vi "Handler - FPGA Health Alert.vi"(8 "error in (no error)":errorcluster, 11 "FPGA Health Info":T1) -> (0 "error out":errorcluster, 3 "Exit?":bool)   [LabVIEW 2018]
uses:
  Top Level/Shared Controls/FPGA Alert Info.ctl
  Error Handler.lvlib
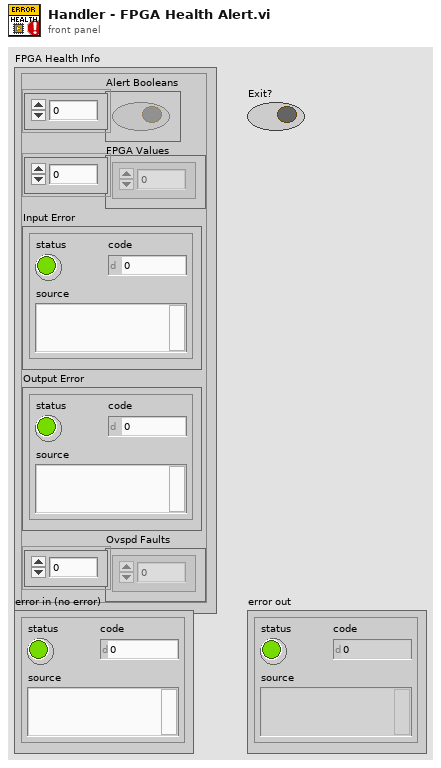
[diagram p1: front panel]
types:
  T1 = typedef "FPGA Alert Info.ctl" = cluster{"Alert Booleans":bool[], "FPGA Values":u64[], "Input Error":errorcluster, "Output Error":errorcluster, "Ovspd Faults":sgl[]}
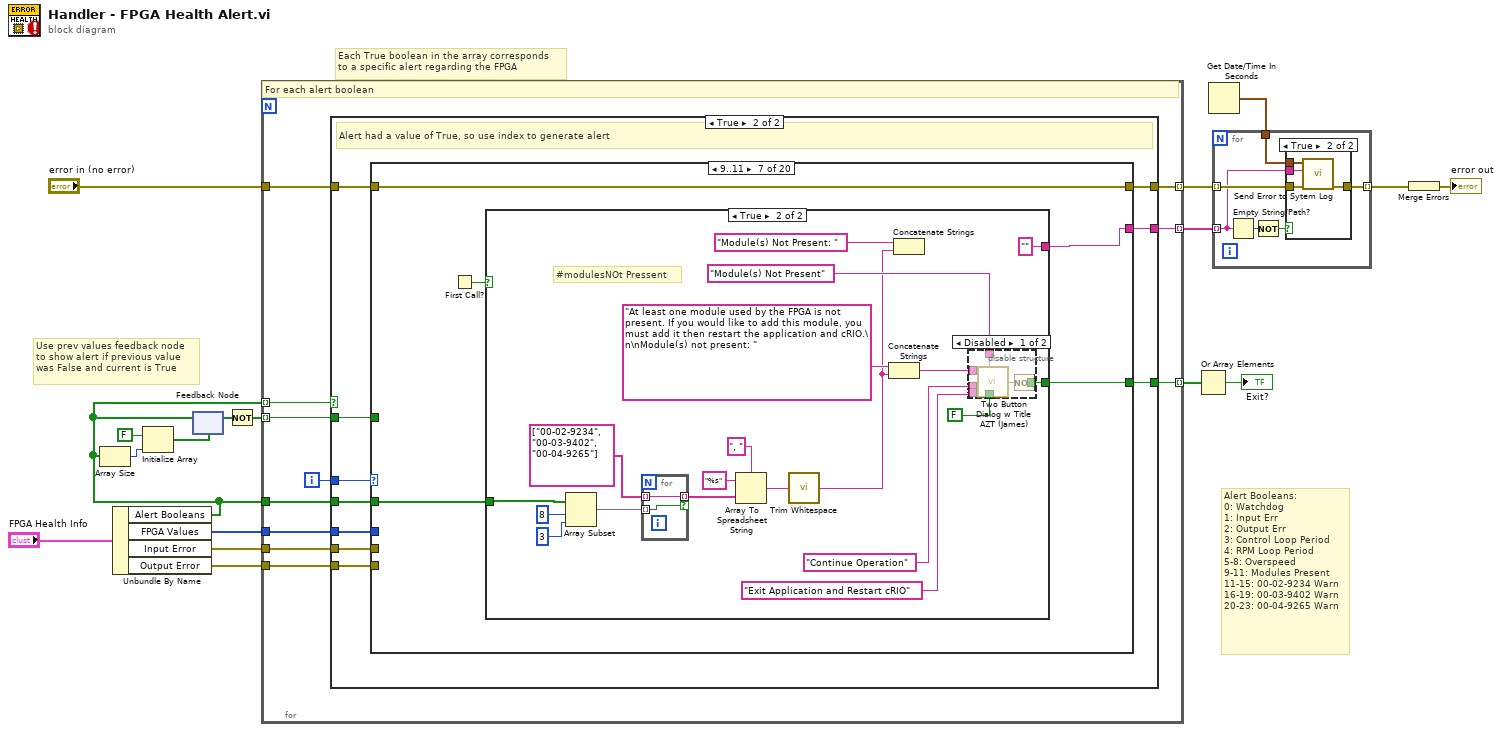
[diagram p0: block diagram]
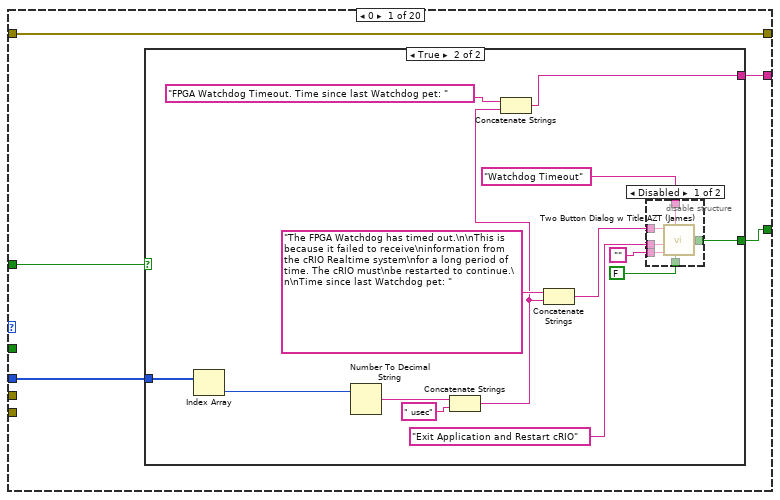
[diagram p4: hidden frame]
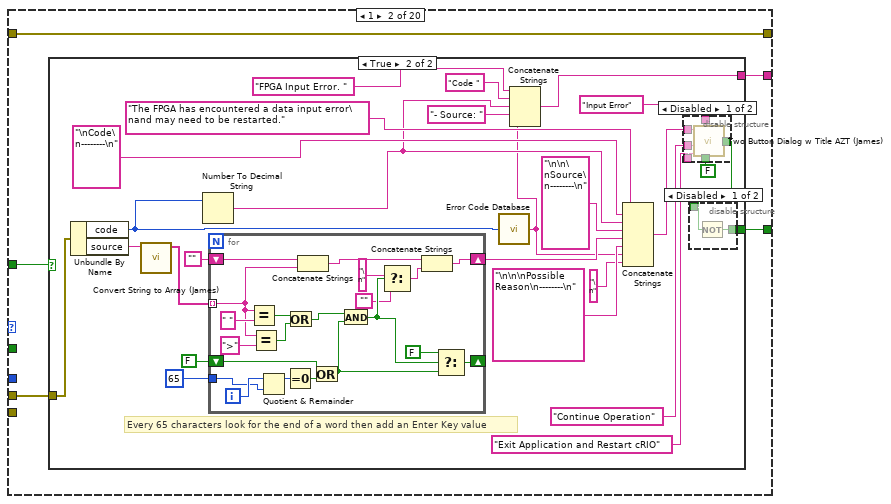
[diagram p7: hidden frame]
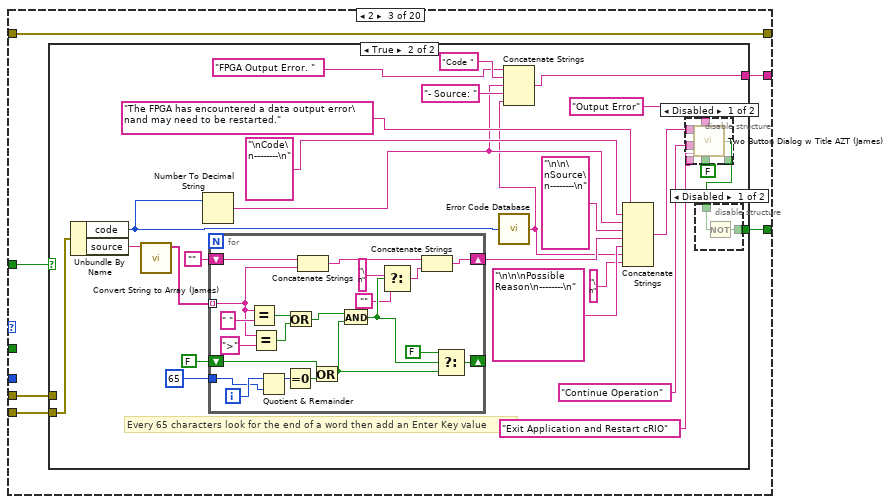
[diagram p11: hidden frame]
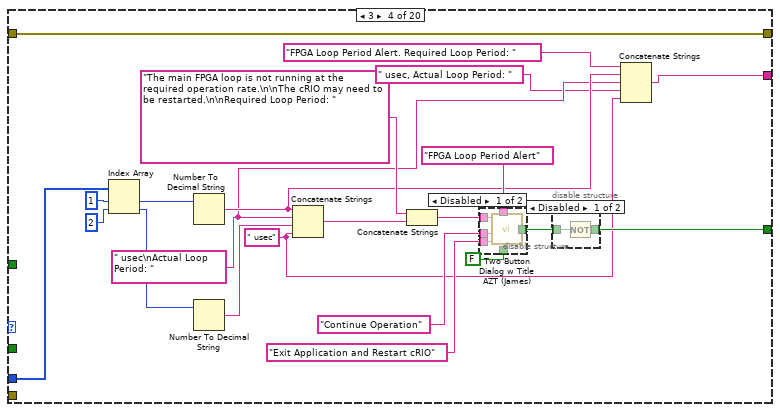
[diagram p15: hidden frame]
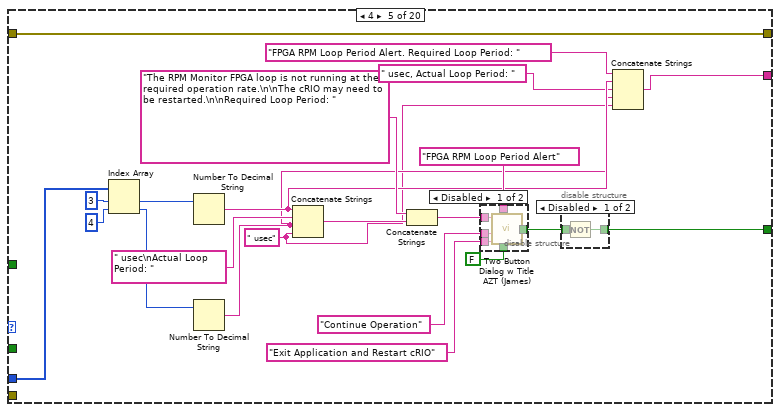
[diagram p18: hidden frame]
diagram:
  # "Alert Booleans:\n0: Watchdog\n1: Input Err\n2: Output Err\n3: Control Loop Period\n4: RPM Loop Period\n5-8: Overspeed\n9-11: Modules Present\n11-15: 00-02-9234 Warn\n16-19: 00-03-9402 Warn\n20-23: 00-04-9265 Warn"
  # "Use prev values feedback node\nto show alert if previous value\nwas False and current is True"
  # "Each True boolean in the array corresponds\nto a specific alert regarding the FPGA"
  n1 = Unbundle By Name("FPGA Health Info") -> ("Alert Booleans"=w9:bool[], "FPGA Values"=w15:u64[], "Input Error"=w12:errorcluster, "Output Error"=w11:errorcluster)
  n2 = Array Size(array=w9) -> (size(s)=w8:i32)
  n3 = Initialize Array(FALSE, w8) -> (w7:bool[])
  n4 = feedback #1(w7) -> (w6:bool[])
  n5 = feedback-in #1(w9) -> ()
  n6 = Not(x=w6) -> (.not. x?=w5:bool[])
  n7 = for {
    tunnel: w9 -> [w28] mode=indexing
    tunnel: "error in (no error)" -> [w26]
    tunnel: [w27] -> w4 mode=indexing
    tunnel: w15 -> [w25]
    tunnel: [w24] -> w16 mode=indexing
    tunnel: w12 -> [w23]
    tunnel: w11 -> [w22]
    tunnel: w9 -> [w21]
    tunnel: w5 -> [w20] mode=indexing
    tunnel: [w19] -> w2 mode=indexing
    i -> [w29]
    # "For each alert boolean"
    n8 = case shown="True" w28 {
      tunnel: w29 -> [_ w40]
      tunnel: [w30 w38] -> w27
      tunnel: w26 -> [w30 w39]
      tunnel: w25 -> [_ w37]
      tunnel: [_ w36] -> w24
      tunnel: w23 -> [_ w35]
      tunnel: w22 -> [_ w34]
      tunnel: w21 -> [_ w33]
      tunnel: w20 -> [_ w32]
      tunnel: [_ w31] -> w19
      frame False {
      }
      frame True {
        # "Alert had a value of True, so use index to generate alert"
        n9 = case shown="9..11" w40 {
          selector: w40 -> [_ _ _ _ _ w249 _ _ _ _ _ _ _ _ _ _ _ _ _ w538]
          tunnel: w39 -> [w45 w70 w131 w207 w237 w251 w278 w309 w328 w347 w366 w385 w404 w423 w442 w462 w481 w501 w520 w545]
          tunnel: [w45 w70 w131 w207 w237 w251 w278 w309 w328 w347 w366 w385 w404 w423 w442 w462 w481 w501 w520 w545] -> w38
          tunnel: w37 -> [w43 _ _ w203 w233 _ _ _ _ _ _ _ _ _ _ _ _ _ _ _]
          tunnel: [w44 w69 w130 w194 w223 w250 w277 w308 w327 w346 w365 w384 w403 w422 w441 w461 w480 w500 w519 _] -> w36
          tunnel: w35 -> [_ w68 w129 _ _ _ _ _ _ _ _ _ _ _ _ _ _ _ _ _]
          tunnel: w34 -> [_ _ w128 _ _ _ _ _ _ _ _ _ _ _ _ _ _ _ _ _]
          tunnel: w33 -> [_ _ _ _ _ _ w275 _ _ _ _ _ _ _ _ _ _ _ _ _]
          tunnel: w32 -> [w42 w67 w127 _ _ w248 _ w307 w326 w345 w364 w383 w402 w421 w440 w460 w479 w499 w518 _]
          tunnel: [w41 w66 w126 w191 w217 w247 w274 _ _ _ _ _ _ _ _ w459 w478 _ _ _] -> w31
          frame 0 {
            n10 = case shown="True" w42 {
              tunnel: [_ w56] -> w44
              tunnel: w43 -> [_ w55]
              tunnel: [_ w46] -> w41
              frame False {
              }
              frame True {
                n11 = Index Array(array=w55) -> (element=w54:u64)  [unwired: 1 in]
                n12 = Number To Decimal String(number=w54) -> (decimal integer string=w53:string)  [unwired: 1 in]
                n13 = Concatenate Strings(w53, " usec" ("string")) -> (w47:string)
                n14 = Concatenate Strings("FPGA Watchdog Timeout. Time since last Watchdog pet: " ("Window Title (\"\")"), w47) -> (w46:string)
                n15 = Concatenate Strings("The FPGA Watchdog has timed out.\n\nThis is because it failed to receive\ninformation from the cRIO Realtime system\nfor a long period of time. The cRIO must\nbe restarted to continue.\n\nTime since last Watchdog pet: " ("message"), w47) -> (w57:string)
                n16 = disable-structure shown="Disabled" {
                  disable-tunnel: "Watchdog Timeout" ("Window Title (\"\")") -> [w65 _]
                  disable-tunnel: w57 -> [w64 _]
                  disable-tunnel: [w63 _] -> w56
                  disable-tunnel: FALSE ("Allow user to close window? (TRUE)") -> [w62 _]
                  disable-tunnel: "Exit Application and Restart cRIO" ("T button name (\"OK\")") -> [w61 _]
                  disable-tunnel: "" -> [w60 _]
                  frame Disabled {
                    n17 = call "Two Button Dialog w Title AZT (James).vi"("Allow user to close window? (TRUE)"=w62, "Window Title (\"\")"=w65, "F button name (\"Cancel\")"=w60, "T button name (\"OK\")"=w61, "message"=w64) -> ("T Button?"=w63:bool)  [unwired: 1 in]
                  }
                  frame Enabled {
                  }
                }
              }
            }
          }
          frame 1 {
            n18 = case shown="True" w67 {
              tunnel: [_ w79] -> w69
              tunnel: w68 -> [_ w82]
              tunnel: [_ w72] -> w66
              frame False {
              }
              frame True {
                # "Every 65 characters look for the end of a word then add an Enter Key value"
                n19 = Unbundle By Name(w82) -> ("code"=w91:i32, "source"=w73:string)
                n20 = call "Convert String to Array (James).vi"("String in"=w73) -> ("Array out"=w88:string[])  [unwired: 9 in, 1 out]
                n21 = Number To Decimal String(number=w91) -> (decimal integer string=w74:string)  [unwired: 1 in]
                n22 = for {
                  tunnel: w88 -> [w119] mode=indexing
                  shift-right: [w116] -> w86
                  shift-left: "" -> [w124]
                  tunnel: 65 ("length") -> [w105]
                  shift-right: [w114] -> _
                  shift-left: FALSE -> [w110]
                  i -> [w106]
                  n23 = Equal?(x=w119, y=" ") -> (x = y?=w120:bool)
                  n24 = Equal?(x=w119, y=">") -> (x = y?=w117:bool)
                  n25 = Quotient & Remainder(x=w106, y=w105) -> (x-y*floor(x/y)=w123:i32)  [unwired: 1 out]
                  n26 = Equal To 0?(x=w123) -> (x = 0?=w122:bool)
                  n27 = Or(x=w120, y=w117) -> (x .or. y?=w111:bool)
                  n28 = Concatenate Strings(w124, w119) -> (w125:string)
                  n29 = Or(x=w110, y=w122) -> (x .or. y?=w109:bool)
                  n30 = And(x=w111, y=w109) -> (x .and. y?=w115:bool)
                  n31 = Select(t="\n", s=w115, f="") -> (s? t:f=w112:string)
                  n32 = Concatenate Strings(w125, w112) -> (w116:string)
                  n33 = Select(t=FALSE, s=w115, f=w109) -> (s? t:f=w114:bool)
                }
                n34 = call <vilib>:"Error Code Database.vi"("Error Code"=w91) -> ("Error Text"=w71:string)
                n35 = Concatenate Strings("FPGA Input Error. " ("Window Title (\"\")"), "Code " ("string"), w74, "- Source: " ("string"), w71) -> (w72:string)
                n36 = Concatenate Strings("The FPGA has encountered a data input error\nand may need to be restarted." ("message"), "\nCode\n--------\n", w74, "\n\n\nSource\n--------\n", w86, "\n\n\nPossible Reason\n--------\n" ("string"), w71, "\n" ("string")) -> (w78:string)
                n37 = disable-structure shown="Disabled" {
                  disable-tunnel: "Input Error" ("Window Title (\"\")") -> [w104 _]
                  disable-tunnel: [w103 _] -> w95
                  disable-tunnel: FALSE ("Allow user to close window? (TRUE)") -> [w102 _]
                  disable-tunnel: w78 -> [w101 _]
                  disable-tunnel: "Continue Operation" ("F button name (\"Cancel\")") -> [w100 _]
                  disable-tunnel: "Exit Application and Restart cRIO" ("T button name (\"OK\")") -> [w99 _]
                  frame Disabled {
                    n38 = call "Two Button Dialog w Title AZT (James).vi"("Allow user to close window? (TRUE)"=w102, "Window Title (\"\")"=w104, "F button name (\"Cancel\")"=w99, "T button name (\"OK\")"=w100, "message"=w101) -> ("T Button?"=w103:bool)  [unwired: 1 in]
                  }
                  frame Enabled {
                  }
                }
                n39 = disable-structure shown="Disabled" {
                  disable-tunnel: w95 -> [w98 _]
                  disable-tunnel: [w97 _] -> w79
                  frame Disabled {
                    n40 = Not(x=w98) -> (.not. x?=w97:bool)
                  }
                  frame Enabled {
                  }
                }
              }
            }
          }
          frame 2 {
            n41 = case shown="True" w127 {
              tunnel: [_ w140] -> w130
              tunnel: w129 -> [_ _]
              tunnel: w128 -> [_ w143]
              tunnel: [_ w136] -> w126
              frame False {
              }
              frame True {
                # "Every 65 characters look for the end of a word then add an Enter Key value"
                n42 = Unbundle By Name(w143) -> ("code"=w152:i32, "source"=w133:string)
                n43 = call "Convert String to Array (James).vi"("String in"=w133) -> ("Array out"=w149:string[])  [unwired: 9 in, 1 out]
                n44 = Number To Decimal String(number=w152) -> (decimal integer string=w134:string)  [unwired: 1 in]
                n45 = for {
                  tunnel: w149 -> [w180] mode=indexing
                  shift-right: [w177] -> w147
                  shift-left: "" -> [w185]
                  tunnel: 65 ("length") -> [w166]
                  shift-right: [w175] -> _
                  shift-left: FALSE -> [w171]
                  i -> [w167]
                  n46 = Equal?(x=w180, y=" ") -> (x = y?=w181:bool)
                  n47 = Equal?(x=w180, y=">") -> (x = y?=w178:bool)
                  n48 = Quotient & Remainder(x=w167, y=w166) -> (x-y*floor(x/y)=w184:i32)  [unwired: 1 out]
                  n49 = Equal To 0?(x=w184) -> (x = 0?=w183:bool)
                  n50 = Or(x=w181, y=w178) -> (x .or. y?=w172:bool)
                  n51 = Concatenate Strings(w185, w180) -> (w186:string)
                  n52 = Or(x=w171, y=w183) -> (x .or. y?=w170:bool)
                  n53 = And(x=w172, y=w170) -> (x .and. y?=w176:bool)
                  n54 = Select(t="\n", s=w176, f="") -> (s? t:f=w173:string)
                  n55 = Concatenate Strings(w186, w173) -> (w177:string)
                  n56 = Select(t=FALSE, s=w176, f=w170) -> (s? t:f=w175:bool)
                }
                n57 = call <vilib>:"Error Code Database.vi"("Error Code"=w152) -> ("Error Text"=w132:string)
                n58 = Concatenate Strings("FPGA Output Error. " ("Window Title (\"\")"), "Code " ("string"), w134, "- Source: " ("string"), w132) -> (w136:string)
                n59 = Concatenate Strings("The FPGA has encountered a data output error\nand may need to be restarted." ("message"), "\nCode\n--------\n", w134, "\n\n\nSource\n--------\n", w147, "\n\n\nPossible Reason\n--------\n" ("string"), w132, "\n" ("string")) -> (w139:string)
                n60 = disable-structure shown="Disabled" {
                  disable-tunnel: "Output Error" ("Window Title (\"\")") -> [w165 _]
                  disable-tunnel: [w164 _] -> w156
                  disable-tunnel: FALSE ("Allow user to close window? (TRUE)") -> [w163 _]
                  disable-tunnel: w139 -> [w162 _]
                  disable-tunnel: "Continue Operation" ("F button name (\"Cancel\")") -> [w161 _]
                  disable-tunnel: "Exit Application and Restart cRIO" ("T button name (\"OK\")") -> [w160 _]
                  frame Disabled {
                    n61 = call "Two Button Dialog w Title AZT (James).vi"("Allow user to close window? (TRUE)"=w163, "Window Title (\"\")"=w165, "F button name (\"Cancel\")"=w160, "T button name (\"OK\")"=w161, "message"=w162) -> ("T Button?"=w164:bool)  [unwired: 1 in]
                  }
                  frame Enabled {
                  }
                }
                n62 = disable-structure shown="Disabled" {
                  disable-tunnel: w156 -> [w159 _]
                  disable-tunnel: [w158 _] -> w140
                  frame Disabled {
                    n63 = Not(x=w159) -> (.not. x?=w158:bool)
                  }
                  frame Enabled {
                  }
                }
              }
            }
          }
          frame 3 {
            w189 = " usec" ("string")
            w190 = " usec\nActual Loop Period: " ("string")
            n64 = Index Array(array=w203, index #1=1 ("index"), index #2=2 ("index")) -> (element #1=w198:u64, element #2=w197:u64)
            n65 = Number To Decimal String(number=w198) -> (decimal integer string=w192:string)  [unwired: 1 in]
            n66 = Number To Decimal String(number=w197) -> (decimal integer string=w188:string)  [unwired: 1 in]
            n67 = Concatenate Strings(w192, w190, w188, w189) -> (w201:string)
            n68 = Concatenate Strings("The main FPGA loop is not running at the required operation rate.\n\nThe cRIO may need to be restarted.\n\nRequired Loop Period: " ("message"), w201) -> (w205:string)
            n69 = disable-structure shown="Disabled" {
              disable-tunnel: "FPGA Loop Period Alert" ("Window Title (\"\")") -> [w216 _]
              disable-tunnel: w205 -> [w215 _]
              disable-tunnel: [w214 _] -> w204
              disable-tunnel: FALSE ("Allow user to close window? (TRUE)") -> [w213 _]
              disable-tunnel: "Continue Operation" ("F button name (\"Cancel\")") -> [w212 _]
              disable-tunnel: "Exit Application and Restart cRIO" ("T button name (\"OK\")") -> [w211 _]
              frame Disabled {
                n70 = call "Two Button Dialog w Title AZT (James).vi"("Allow user to close window? (TRUE)"=w213, "Window Title (\"\")"=w216, "F button name (\"Cancel\")"=w211, "T button name (\"OK\")"=w212, "message"=w215) -> ("T Button?"=w214:bool)  [unwired: 1 in]
              }
              frame Enabled {
              }
            }
            n71 = disable-structure shown="Disabled" {
              disable-tunnel: w204 -> [w210 _]
              disable-tunnel: [w209 _] -> w194
              frame Disabled {
                n72 = Not(x=w210) -> (.not. x?=w209:bool)
              }
              frame Enabled {
              }
            }
            n73 = Concatenate Strings("FPGA Loop Period Alert. Required Loop Period: " ("Window Title (\"\")"), w192, w190, " usec, Actual Loop Period: " ("string"), w189) -> (w191:string)
          }
          frame 4 {
            w218 = " usec" ("string")
            n74 = Index Array(array=w233, index #1=3 ("index"), index #2=4 ("index")) -> (element #1=w228:u64, element #2=w227:u64)
            n75 = Number To Decimal String(number=w228) -> (decimal integer string=w221:string)  [unwired: 1 in]
            n76 = Number To Decimal String(number=w227) -> (decimal integer string=w219:string)  [unwired: 1 in]
            n77 = Concatenate Strings(w221, " usec\nActual Loop Period: " ("string"), w219, w218) -> (w231:string)
            n78 = Concatenate Strings("The RPM Monitor FPGA loop is not running at the required operation rate.\n\nThe cRIO may need to be restarted.\n\nRequired Loop Period: " ("message"), w231) -> (w235:string)
            n79 = disable-structure shown="Disabled" {
              disable-tunnel: "FPGA RPM Loop Period Alert" ("Window Title (\"\")") -> [w246 _]
              disable-tunnel: w235 -> [w245 _]
              disable-tunnel: [w244 _] -> w234
              disable-tunnel: FALSE ("Allow user to close window? (TRUE)") -> [w243 _]
              disable-tunnel: "Continue Operation" ("F button name (\"Cancel\")") -> [w242 _]
              disable-tunnel: "Exit Application and Restart cRIO" ("T button name (\"OK\")") -> [w241 _]
              frame Disabled {
                n80 = call "Two Button Dialog w Title AZT (James).vi"("Allow user to close window? (TRUE)"=w243, "Window Title (\"\")"=w246, "F button name (\"Cancel\")"=w241, "T button name (\"OK\")"=w242, "message"=w245) -> ("T Button?"=w244:bool)  [unwired: 1 in]
              }
              frame Enabled {
              }
            }
            n81 = disable-structure shown="Disabled" {
              disable-tunnel: w234 -> [w240 _]
              disable-tunnel: [w239 _] -> w223
              frame Disabled {
                n82 = Not(x=w240) -> (.not. x?=w239:bool)
              }
              frame Enabled {
              }
            }
            n83 = Concatenate Strings("FPGA RPM Loop Period Alert. Required Loop Period: " ("Window Title (\"\")"), w221, " usec, Actual Loop Period: " ("string"), w219, w218) -> (w217:string)
          }
          frame 5..8 {
            n84 = case shown="True" w248 {
              tunnel: [_ w255] -> w250
              tunnel: w249 -> [_ w259]
              tunnel: [_ w252] -> w247
              frame False {
              }
              frame True {
                n85 = Subtract(x=w259, y=4) -> (x-y=w260:i32)
                n86 = Number To Decimal String(number=w260) -> (decimal integer string=w253:string)  [unwired: 1 in]
                n87 = Concatenate Strings("The FPGA has indicated an Overspeed Fault.\n\nFault Index: " ("message"), w253) -> (w263:string)
                n88 = Concatenate Strings("Overspeed Fault. Fault Index: " ("Window Title (\"\")"), w253) -> (w252:string)
                n89 = disable-structure shown="Disabled" {
                  disable-tunnel: "Overspeed Fault" ("Window Title (\"\")") -> [w273 _]
                  disable-tunnel: w263 -> [w272 _]
                  disable-tunnel: [w271 _] -> w262
                  disable-tunnel: FALSE ("Allow user to close window? (TRUE)") -> [w270 _]
                  disable-tunnel: "Continue Operation" ("F button name (\"Cancel\")") -> [w269 _]
                  disable-tunnel: "Exit Application and Restart cRIO" ("T button name (\"OK\")") -> [w268 _]
                  frame Disabled {
                    n90 = call "Two Button Dialog w Title AZT (James).vi"("Allow user to close window? (TRUE)"=w270, "Window Title (\"\")"=w273, "F button name (\"Cancel\")"=w268, "T button name (\"OK\")"=w269, "message"=w272) -> ("T Button?"=w271:bool)  [unwired: 1 in]
                  }
                  frame Enabled {
                  }
                }
                n91 = disable-structure shown="Disabled" {
                  disable-tunnel: w262 -> [w267 _]
                  disable-tunnel: [w266 _] -> w255
                  frame Disabled {
                    n92 = Not(x=w267) -> (.not. x?=w266:bool)
                  }
                  frame Enabled {
                  }
                }
              }
            }
          }
          frame 9..11 {
            n93 = First Call?() -> (First Call?: T/F=w276:bool)
            n94 = case shown="True" w276 {
              tunnel: [_ w283] -> w277
              tunnel: w275 -> [_ w280]
              tunnel: [_ "" ("String")] -> w274
              frame False {
              }
              frame True {
                # "#modulesNOt Pressent"
                n95 = Array Subset(array=w280, index=8, length=3) -> (w291:bool[])
                n96 = for {
                  tunnel: w291 -> [w305] mode=indexing
                  tunnel: string[] ["00-02-9234", "00-03-9402", "00-04-9265"] -> [w306] mode=indexing
                  tunnel: [w306] -> w289 mode=indexing if=w305
                }
                n97 = Array To Spreadsheet String(delimiter (Tab)=", ", array=w289, 3:"%s" ("format string")) -> (spreadsheet string=w287:string)
                n98 = call <vilib>:"Trim Whitespace.vi"("string"=w287) -> ("trimmed string"=w281:string)  [unwired: 1 in]
                n99 = Concatenate Strings("At least one module used by the FPGA is not present. If you would like to add this module, you must add it then restart the application and cRIO.\n\nModule(s) not present: " ("message"), w281) -> (w295:string)
                n100 = Concatenate Strings("Module(s) Not Present: " ("Window Title (\"\")"), w281) -> ()  [unwired: 1 out]
                n101 = disable-structure shown="Disabled" {
                  disable-tunnel: "Module(s) Not Present" ("Window Title (\"\")") -> [w304 _]
                  disable-tunnel: w295 -> [w303 _]
                  disable-tunnel: FALSE ("Allow user to close window? (TRUE)") -> [w301 _]
                  disable-tunnel: "Continue Operation" ("F button name (\"Cancel\")") -> [w300 _]
                  disable-tunnel: "Exit Application and Restart cRIO" ("T button name (\"OK\")") -> [w299 _]
                  disable-tunnel: [w298 _] -> w283
                  frame Disabled {
                    n102 = call "Two Button Dialog w Title AZT (James).vi"("Allow user to close window? (TRUE)"=w301, "Window Title (\"\")"=w304, "F button name (\"Cancel\")"=w299, "T button name (\"OK\")"=w300, "message"=w303) -> ("T Button?"=w302:bool)  [unwired: 1 in]
                    n103 = Not(x=w302) -> (.not. x?=w298:bool)
                  }
                  frame Enabled {
                  }
                }
              }
            }
          }
          frame 12 {
            n104 = case shown="True" w307 {
              tunnel: [_ w310] -> w308
              frame False {
              }
              frame True {
                n105 = Concatenate Strings("" ("message")) -> (w315:string)
                n106 = disable-structure shown="Disabled" {
                  disable-tunnel: "Unused 00-02-9234 Warning" ("Window Title (\"\")") -> [w325 _]
                  disable-tunnel: w315 -> [w324 _]
                  disable-tunnel: [w323 _] -> w314
                  disable-tunnel: FALSE ("Allow user to close window? (TRUE)") -> [w322 _]
                  disable-tunnel: "Continue Operation" ("F button name (\"Cancel\")") -> [w321 _]
                  disable-tunnel: "Exit Application and Restart cRIO" ("T button name (\"OK\")") -> [w320 _]
                  frame Disabled {
                    n107 = call "Two Button Dialog w Title AZT (James).vi"("Allow user to close window? (TRUE)"=w322, "Window Title (\"\")"=w325, "F button name (\"Cancel\")"=w320, "T button name (\"OK\")"=w321, "message"=w324) -> ("T Button?"=w323:bool)  [unwired: 1 in]
                  }
                  frame Enabled {
                  }
                }
                n108 = disable-structure shown="Disabled" {
                  disable-tunnel: w314 -> [w319 _]
                  disable-tunnel: [w318 _] -> w310
                  frame Disabled {
                    n109 = Not(x=w319) -> (.not. x?=w318:bool)
                  }
                  frame Enabled {
                  }
                }
              }
            }
          }
          frame 13 {
            n110 = case shown="True" w326 {
              tunnel: [_ w329] -> w327
              frame False {
              }
              frame True {
                n111 = Concatenate Strings("" ("message")) -> (w334:string)
                n112 = disable-structure shown="Disabled" {
                  disable-tunnel: "Unused 00-02-9234 Warning" ("Window Title (\"\")") -> [w344 _]
                  disable-tunnel: w334 -> [w343 _]
                  disable-tunnel: [w342 _] -> w333
                  disable-tunnel: FALSE ("Allow user to close window? (TRUE)") -> [w341 _]
                  disable-tunnel: "Continue Operation" ("F button name (\"Cancel\")") -> [w340 _]
                  disable-tunnel: "Exit Application and Restart cRIO" ("T button name (\"OK\")") -> [w339 _]
                  frame Disabled {
                    n113 = call "Two Button Dialog w Title AZT (James).vi"("Allow user to close window? (TRUE)"=w341, "Window Title (\"\")"=w344, "F button name (\"Cancel\")"=w339, "T button name (\"OK\")"=w340, "message"=w343) -> ("T Button?"=w342:bool)  [unwired: 1 in]
                  }
                  frame Enabled {
                  }
                }
                n114 = disable-structure shown="Disabled" {
                  disable-tunnel: w333 -> [w338 _]
                  disable-tunnel: [w337 _] -> w329
                  frame Disabled {
                    n115 = Not(x=w338) -> (.not. x?=w337:bool)
                  }
                  frame Enabled {
                  }
                }
              }
            }
          }
          frame 14 {
            n116 = case shown="True" w345 {
              tunnel: [_ w348] -> w346
              frame False {
              }
              frame True {
                n117 = Concatenate Strings("" ("message")) -> (w353:string)
                n118 = disable-structure shown="Disabled" {
                  disable-tunnel: "Unused 00-02-9234 Warning" ("Window Title (\"\")") -> [w363 _]
                  disable-tunnel: w353 -> [w362 _]
                  disable-tunnel: [w361 _] -> w352
                  disable-tunnel: FALSE ("Allow user to close window? (TRUE)") -> [w360 _]
                  disable-tunnel: "Continue Operation" ("F button name (\"Cancel\")") -> [w359 _]
                  disable-tunnel: "Exit Application and Restart cRIO" ("T button name (\"OK\")") -> [w358 _]
                  frame Disabled {
                    n119 = call "Two Button Dialog w Title AZT (James).vi"("Allow user to close window? (TRUE)"=w360, "Window Title (\"\")"=w363, "F button name (\"Cancel\")"=w358, "T button name (\"OK\")"=w359, "message"=w362) -> ("T Button?"=w361:bool)  [unwired: 1 in]
                  }
                  frame Enabled {
                  }
                }
                n120 = disable-structure shown="Disabled" {
                  disable-tunnel: w352 -> [w357 _]
                  disable-tunnel: [w356 _] -> w348
                  frame Disabled {
                    n121 = Not(x=w357) -> (.not. x?=w356:bool)
                  }
                  frame Enabled {
                  }
                }
              }
            }
          }
          frame 15 {
            n122 = case shown="True" w364 {
              tunnel: [_ w367] -> w365
              frame False {
              }
              frame True {
                n123 = Concatenate Strings("" ("message")) -> (w372:string)
                n124 = disable-structure shown="Disabled" {
                  disable-tunnel: "Unused 00-02-9234 Warning" ("Window Title (\"\")") -> [w382 _]
                  disable-tunnel: w372 -> [w381 _]
                  disable-tunnel: [w380 _] -> w371
                  disable-tunnel: FALSE ("Allow user to close window? (TRUE)") -> [w379 _]
                  disable-tunnel: "Continue Operation" ("F button name (\"Cancel\")") -> [w378 _]
                  disable-tunnel: "Exit Application and Restart cRIO" ("T button name (\"OK\")") -> [w377 _]
                  frame Disabled {
                    n125 = call "Two Button Dialog w Title AZT (James).vi"("Allow user to close window? (TRUE)"=w379, "Window Title (\"\")"=w382, "F button name (\"Cancel\")"=w377, "T button name (\"OK\")"=w378, "message"=w381) -> ("T Button?"=w380:bool)  [unwired: 1 in]
                  }
                  frame Enabled {
                  }
                }
                n126 = disable-structure shown="Disabled" {
                  disable-tunnel: w371 -> [w376 _]
                  disable-tunnel: [w375 _] -> w367
                  frame Disabled {
                    n127 = Not(x=w376) -> (.not. x?=w375:bool)
                  }
                  frame Enabled {
                  }
                }
              }
            }
          }
          frame 16 {
            n128 = case shown="True" w383 {
              tunnel: [_ w386] -> w384
              frame False {
              }
              frame True {
                n129 = Concatenate Strings("" ("message")) -> (w391:string)
                n130 = disable-structure shown="Disabled" {
                  disable-tunnel: "Unused 00-03-9402 Warning" ("Window Title (\"\")") -> [w401 _]
                  disable-tunnel: w391 -> [w400 _]
                  disable-tunnel: [w399 _] -> w390
                  disable-tunnel: FALSE ("Allow user to close window? (TRUE)") -> [w398 _]
                  disable-tunnel: "Exit Application and Restart cRIO" ("T button name (\"OK\")") -> [w397 _]
                  disable-tunnel: "Continue Operation" ("F button name (\"Cancel\")") -> [w396 _]
                  frame Disabled {
                    n131 = call "Two Button Dialog w Title AZT (James).vi"("Allow user to close window? (TRUE)"=w398, "Window Title (\"\")"=w401, "F button name (\"Cancel\")"=w397, "T button name (\"OK\")"=w396, "message"=w400) -> ("T Button?"=w399:bool)  [unwired: 1 in]
                  }
                  frame Enabled {
                  }
                }
                n132 = disable-structure shown="Disabled" {
                  disable-tunnel: w390 -> [w395 _]
                  disable-tunnel: [w394 _] -> w386
                  frame Disabled {
                    n133 = Not(x=w395) -> (.not. x?=w394:bool)
                  }
                  frame Enabled {
                  }
                }
              }
            }
          }
          frame 17 {
            n134 = case shown="True" w402 {
              tunnel: [_ w407] -> w403
              frame False {
              }
              frame True {
                n135 = Concatenate Strings("" ("message")) -> (w410:string)
                n136 = disable-structure shown="Disabled" {
                  disable-tunnel: "Unused 00-03-9402 Warning" ("Window Title (\"\")") -> [w420 _]
                  disable-tunnel: w410 -> [w419 _]
                  disable-tunnel: [w418 _] -> w409
                  disable-tunnel: FALSE ("Allow user to close window? (TRUE)") -> [w417 _]
                  disable-tunnel: "Continue Operation" ("F button name (\"Cancel\")") -> [w416 _]
                  disable-tunnel: "Exit Application and Restart cRIO" ("T button name (\"OK\")") -> [w415 _]
                  frame Disabled {
                    n137 = call "Two Button Dialog w Title AZT (James).vi"("Allow user to close window? (TRUE)"=w417, "Window Title (\"\")"=w420, "F button name (\"Cancel\")"=w415, "T button name (\"OK\")"=w416, "message"=w419) -> ("T Button?"=w418:bool)  [unwired: 1 in]
                  }
                  frame Enabled {
                  }
                }
                n138 = disable-structure shown="Disabled" {
                  disable-tunnel: w409 -> [w414 _]
                  disable-tunnel: [w413 _] -> w407
                  frame Disabled {
                    n139 = Not(x=w414) -> (.not. x?=w413:bool)
                  }
                  frame Enabled {
                  }
                }
              }
            }
          }
          frame 18 {
            n140 = case shown="True" w421 {
              tunnel: [_ w424] -> w422
              frame False {
              }
              frame True {
                n141 = Concatenate Strings("" ("message")) -> (w429:string)
                n142 = disable-structure shown="Disabled" {
                  disable-tunnel: "Unused 00-03-9402 Warning" ("Window Title (\"\")") -> [w439 _]
                  disable-tunnel: w429 -> [w438 _]
                  disable-tunnel: [w437 _] -> w428
                  disable-tunnel: FALSE ("Allow user to close window? (TRUE)") -> [w436 _]
                  disable-tunnel: "Continue Operation" ("F button name (\"Cancel\")") -> [w435 _]
                  disable-tunnel: "Exit Application and Restart cRIO" ("T button name (\"OK\")") -> [w434 _]
                  frame Disabled {
                    n143 = call "Two Button Dialog w Title AZT (James).vi"("Allow user to close window? (TRUE)"=w436, "Window Title (\"\")"=w439, "F button name (\"Cancel\")"=w434, "T button name (\"OK\")"=w435, "message"=w438) -> ("T Button?"=w437:bool)  [unwired: 1 in]
                  }
                  frame Enabled {
                  }
                }
                n144 = disable-structure shown="Disabled" {
                  disable-tunnel: w428 -> [w433 _]
                  disable-tunnel: [w432 _] -> w424
                  frame Disabled {
                    n145 = Not(x=w433) -> (.not. x?=w432:bool)
                  }
                  frame Enabled {
                  }
                }
              }
            }
          }
          frame 19 {
            n146 = case shown="True" w440 {
              tunnel: [_ w443] -> w441
              frame False {
              }
              frame True {
                n147 = Concatenate Strings("" ("message")) -> (w448:string)
                n148 = disable-structure shown="Disabled" {
                  disable-tunnel: "Unused 00-03-9402 Warning" ("Window Title (\"\")") -> [w458 _]
                  disable-tunnel: w448 -> [w457 _]
                  disable-tunnel: [w456 _] -> w447
                  disable-tunnel: FALSE ("Allow user to close window? (TRUE)") -> [w455 _]
                  disable-tunnel: "Continue Operation" ("F button name (\"Cancel\")") -> [w454 _]
                  disable-tunnel: "Exit Application and Restart cRIO" ("T button name (\"OK\")") -> [w453 _]
                  frame Disabled {
                    n149 = call "Two Button Dialog w Title AZT (James).vi"("Allow user to close window? (TRUE)"=w455, "Window Title (\"\")"=w458, "F button name (\"Cancel\")"=w453, "T button name (\"OK\")"=w454, "message"=w457) -> ("T Button?"=w456:bool)  [unwired: 1 in]
                  }
                  frame Enabled {
                  }
                }
                n150 = disable-structure shown="Disabled" {
                  disable-tunnel: w447 -> [w452 _]
                  disable-tunnel: [w451 _] -> w443
                  frame Disabled {
                    n151 = Not(x=w452) -> (.not. x?=w451:bool)
                  }
                  frame Enabled {
                  }
                }
              }
            }
          }
          frame 20 {
            n152 = case shown="True" w460 {
              tunnel: [_ w465] -> w461
              tunnel: [_ "00-04-9265 Output Warning - Code 65543. Power supply voltage out of range." ("Window Title (\"\")")] -> w459
              frame False {
              }
              frame True {
                n153 = Concatenate Strings("00-04-9265 Output Warning - Code 65543\n\nThe power supply voltage level is out of range.\n            Check the supply voltage and the module connections.\n" ("message")) -> (w469:string)
                n154 = disable-structure shown="Disabled" {
                  disable-tunnel: w469 -> [w477 _]
                  disable-tunnel: FALSE ("Allow user to close window? (TRUE)") -> [w475 _]
                  disable-tunnel: "Continue Operation" ("F button name (\"Cancel\")") -> [w474 _]
                  disable-tunnel: "Exit Application and Restart cRIO" ("T button name (\"OK\")") -> [w473 _]
                  disable-tunnel: [w472 _] -> w465
                  disable-tunnel: "00-04-9265 Output Warning" ("Window Title (\"\")") -> [w471 _]
                  frame Disabled {
                    n155 = call "Two Button Dialog w Title AZT (James).vi"("Allow user to close window? (TRUE)"=w475, "Window Title (\"\")"=w471, "F button name (\"Cancel\")"=w473, "T button name (\"OK\")"=w474, "message"=w477) -> ("T Button?"=w476:bool)  [unwired: 1 in]
                    n156 = Not(x=w476) -> (.not. x?=w472:bool)
                  }
                  frame Enabled {
                  }
                }
              }
            }
          }
          frame 21 {
            n157 = case shown="True" w479 {
              tunnel: [_ w485] -> w480
              tunnel: [_ "00-04-9265 Output Warning - Code 65542. Open current loop on one or more channels." ("Window Title (\"\")")] -> w478
              frame False {
              }
              frame True {
                n158 = Concatenate Strings("00-04-9265 Output Warning - Code 65542\n\nOne or more channels have detected an open current loop. Check the module connections.\n" ("message")) -> (w488:string)
                n159 = disable-structure shown="Disabled" {
                  disable-tunnel: "00-04-9265 Output Warning" ("Window Title (\"\")") -> [w498 _]
                  disable-tunnel: w488 -> [w497 _]
                  disable-tunnel: "Continue Operation" ("F button name (\"Cancel\")") -> [w496 _]
                  disable-tunnel: "Exit Application and Restart cRIO" ("T button name (\"OK\")") -> [w495 _]
                  disable-tunnel: [w494 _] -> w484
                  disable-tunnel: FALSE ("Allow user to close window? (TRUE)") -> [w493 _]
                  frame Disabled {
                    n160 = call "Two Button Dialog w Title AZT (James).vi"("Allow user to close window? (TRUE)"=w493, "Window Title (\"\")"=w498, "F button name (\"Cancel\")"=w495, "T button name (\"OK\")"=w496, "message"=w497) -> ("T Button?"=w494:bool)  [unwired: 1 in]
                  }
                  frame Enabled {
                  }
                }
                n161 = disable-structure shown="Disabled" {
                  disable-tunnel: [w492 _] -> w485
                  disable-tunnel: w484 -> [w491 _]
                  frame Disabled {
                    n162 = Not(x=w491) -> (.not. x?=w492:bool)
                  }
                  frame Enabled {
                  }
                }
              }
            }
          }
          frame 22 {
            n163 = case shown="True" w499 {
              tunnel: [_ w502] -> w500
              frame False {
              }
              frame True {
                n164 = Concatenate Strings("" ("message")) -> (w507:string)
                n165 = disable-structure shown="Disabled" {
                  disable-tunnel: "Unused 00-04-9265 Warning" ("Window Title (\"\")") -> [w517 _]
                  disable-tunnel: w507 -> [w516 _]
                  disable-tunnel: [w515 _] -> w506
                  disable-tunnel: FALSE ("Allow user to close window? (TRUE)") -> [w514 _]
                  disable-tunnel: "Continue Operation" ("F button name (\"Cancel\")") -> [w513 _]
                  disable-tunnel: "Exit Application and Restart cRIO" ("T button name (\"OK\")") -> [w512 _]
                  frame Disabled {
                    n166 = call "Two Button Dialog w Title AZT (James).vi"("Allow user to close window? (TRUE)"=w514, "Window Title (\"\")"=w517, "F button name (\"Cancel\")"=w512, "T button name (\"OK\")"=w513, "message"=w516) -> ("T Button?"=w515:bool)  [unwired: 1 in]
                  }
                  frame Enabled {
                  }
                }
                n167 = disable-structure shown="Disabled" {
                  disable-tunnel: w506 -> [w511 _]
                  disable-tunnel: [w510 _] -> w502
                  frame Disabled {
                    n168 = Not(x=w511) -> (.not. x?=w510:bool)
                  }
                  frame Enabled {
                  }
                }
              }
            }
          }
          frame 23 {
            n169 = case shown="True" w518 {
              tunnel: [_ w521] -> w519
              frame False {
              }
              frame True {
                n170 = Concatenate Strings("" ("message")) -> (w526:string)
                n171 = disable-structure shown="Disabled" {
                  disable-tunnel: "Unused 00-04-9265 Warning" ("Window Title (\"\")") -> [w536 _]
                  disable-tunnel: w526 -> [w535 _]
                  disable-tunnel: [w534 _] -> w525
                  disable-tunnel: FALSE ("Allow user to close window? (TRUE)") -> [w533 _]
                  disable-tunnel: "Continue Operation" ("F button name (\"Cancel\")") -> [w532 _]
                  disable-tunnel: "Exit Application and Restart cRIO" ("T button name (\"OK\")") -> [w531 _]
                  frame Disabled {
                    n172 = call "Two Button Dialog w Title AZT (James).vi"("Allow user to close window? (TRUE)"=w533, "Window Title (\"\")"=w536, "F button name (\"Cancel\")"=w531, "T button name (\"OK\")"=w532, "message"=w535) -> ("T Button?"=w534:bool)  [unwired: 1 in]
                  }
                  frame Enabled {
                  }
                }
                n173 = disable-structure shown="Disabled" {
                  disable-tunnel: w525 -> [w530 _]
                  disable-tunnel: [w529 _] -> w521
                  frame Disabled {
                    n174 = Not(x=w530) -> (.not. x?=w529:bool)
                  }
                  frame Enabled {
                  }
                }
              }
            }
          }
          frame Default {
            n175 = Number To Decimal String(number=w538) -> (decimal integer string=w542:string)  [unwired: 1 in]
            n176 = Concatenate Strings(" " ("string"), w542) -> (w540:string)
            n177 = Concatenate Strings("There has been an unhandled FPGA Alert.\n\nAlert index:" ("message"), w540) -> (w543:string)
            n178 = disable-structure shown="Disabled" {
              disable-tunnel: "Unhandled FPGA Alert" ("Window Title (\"\")") -> [w550 _]
              disable-tunnel: w543 -> [w549 _]
              disable-tunnel: FALSE ("Allow user to close window? (TRUE)") -> [w548 _]
              disable-tunnel: "Continue" ("T button name (\"OK\")") -> [w547 _]
              frame Disabled {
                n179 = call "Two Button Dialog w Title AZT (James).vi"("Allow user to close window? (TRUE)"=w548, "Window Title (\"\")"=w550, "T button name (\"OK\")"=w547, "message"=w549) -> ()  [unwired: 2 in, 1 out]
              }
              frame Enabled {
              }
            }
          }
        }
      }
    }
  }
  n180 = Or Array Elements(Boolean array=w16) -> (logical OR=→"Exit?":bool)
  n181 = Get Date/Time In Seconds() -> (seconds since 1Jan1904=w1:timestamp)
  n182 = for {
    tunnel: w4 -> [w556] mode=indexing
    tunnel: [w555] -> w3 mode=indexing
    tunnel: w2 -> [w552] mode=indexing
    tunnel: w1 -> [w551]
    n183 = Empty String/Path?(string/path=w552) -> (empty?=w554:bool)
    n184 = Not(x=w554) -> (.not. x?=w553:bool)
    n185 = case shown="True" w553 {
      tunnel: w556 -> [w557 w561]
      tunnel: [w557 w560] -> w555
      tunnel: w552 -> [_ w559]
      tunnel: w551 -> [_ w558]
      frame False {
      }
      frame True {
        n186 = call "Send Error to Sytem Log.vi"("error in (no error)"=w561, "Error Title or Message"=w559, "Timestamp"=w558) -> ("error out"=w560:errorcluster)  [unwired: 8 in]
      }
    }
  }
  n187 = Merge Errors(w3) -> (→"error out":errorcluster)
